vi "Scriptsaver2012.vi"(2 "Filename":string, 3 "Save (0)/Load (1)":bool, 4 "Script":string) -> (0 "File not found":bool, 1 "Loaded Script":string)   [LabVIEW 2012]
panel:
  # "If set to save or if specified file does not exist, Loaded Script returns\nan empty string."
  # "Will neither save nor load anything if filename empty"
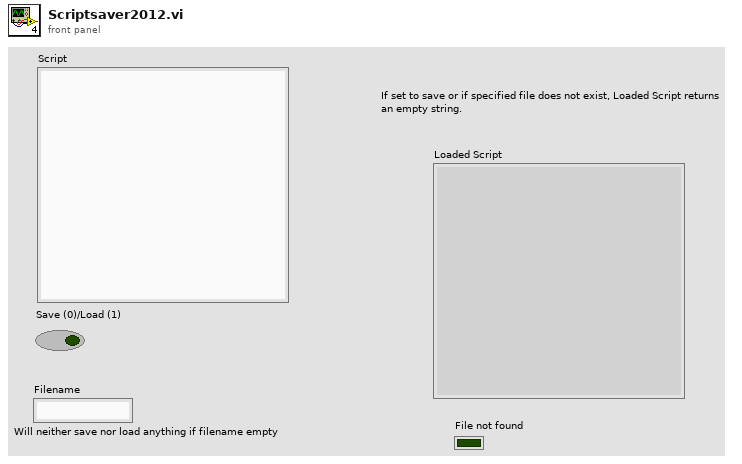
[diagram p1: front panel]
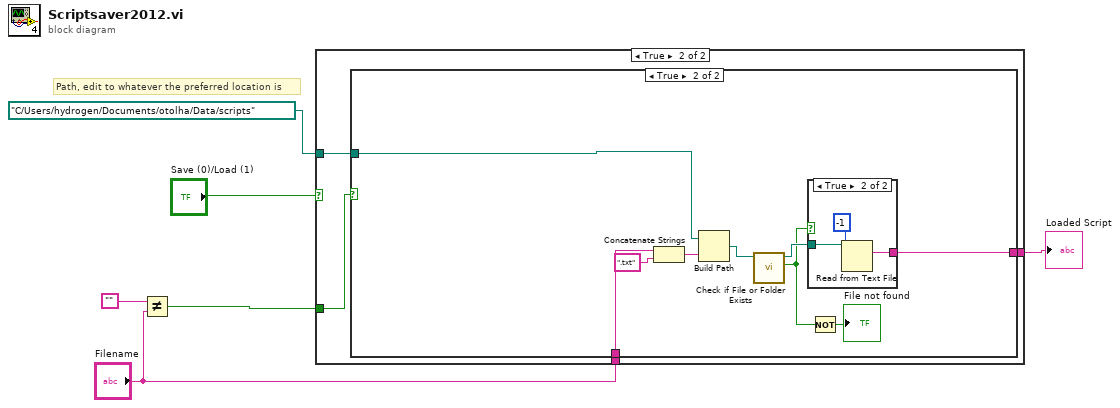
[diagram p0: block diagram]
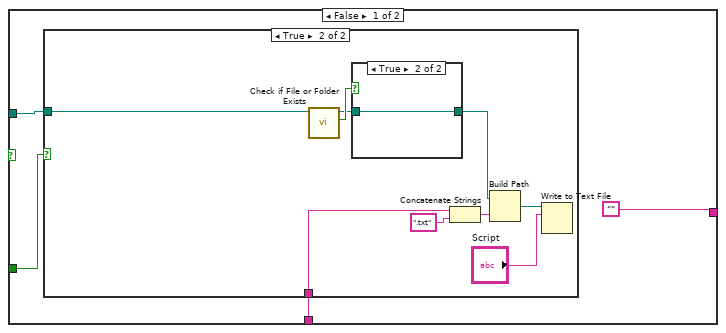
[diagram p2: hidden frame]
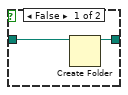
[diagram p4: hidden frame]
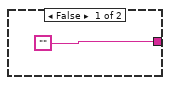
[diagram p5: hidden frame]
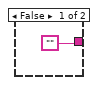
[diagram p6: hidden frame]
diagram:
  # "Path, edit to whatever the preferred location is"
  n1 = Not Equal?(x="", y="Filename") -> (x != y?=w4:bool)
  n2 = case shown="True" "Save (0)/Load (1)" {
    tunnel: "Filename" -> [w10 w26]
    tunnel: w4 -> [w9 w25]
    tunnel: ["" w24] -> w2
    tunnel: path "C:/Users/hydrogen/Documents/otolha/Data/scripts" ("base path") -> [w7 w23]
    frame False {
      n3 = case shown="True" w9 {
        tunnel: w10 -> [_ w15]
        tunnel: w7 -> [_ w12]
        frame False {
        }
        frame True {
          n4 = call <vilib>:"Check if File or Folder Exists.vi"("path"=w12) -> ("file or folder exists?"=w16:bool, "dup path"=w11:path)  [unwired: 8 in, 1 out]
          n5 = case shown="True" w16 {
            tunnel: w11 -> [w21 w22]
            tunnel: [w20 w22] -> w17
            frame False {
              n6 = Create Folder(path (use dialog)=w21) -> (created path=w20:path)  [unwired: 2 in, 2 out]
            }
            frame True {
            }
          }
          n7 = Concatenate Strings(w15, ".txt" ("string")) -> (w13:string)
          n8 = Build Path(base path=w17, name or relative path=w13) -> (appended path=w18:path)
          n9 = Write to Text File(file (use dialog)=w18, text="Script") -> ()  [unwired: 2 in, 3 out]
        }
      }
    }
    frame True {
      n10 = case shown="True" w25 {
        tunnel: w26 -> [_ w36]
        tunnel: ["" w33] -> w24
        tunnel: w23 -> [_ w32]
        frame False {
        }
        frame True {
          n11 = Concatenate Strings(w36, ".txt" ("string")) -> (w34:string)
          n12 = Build Path(base path=w32, name or relative path=w34) -> (appended path=w31:path)
          n13 = call <vilib>:"Check if File or Folder Exists.vi"("path"=w31) -> ("file or folder exists?"=w28:bool, "dup path"=w30:path)  [unwired: 8 in, 1 out]
          n14 = case shown="True" w28 {
            tunnel: ["" w39] -> w33
            tunnel: w30 -> [_ w38]
            frame False {
            }
            frame True {
              n15 = Read from Text File(file (use dialog)=w38, count=-1) -> (text=w39:string)  [unwired: 2 in, 3 out]
            }
          }
          n16 = Not(x=w28) -> (.not. x?=→"File not found":bool)
        }
      }
    }
  }
  "Loaded Script" <- w2
